vi "Current EXE File Path.vi"(8 "error in (no error)":errorcluster) -> (0 "error out":errorcluster, 3 "Current EXE Path":path)   [LabVIEW 2016, in "SLL Application.lvlib"]
doc: "Provides the current EXE file path. \n\nThis will not work in LabVIEW development environment."
uses:
  SLL Application.lvlib
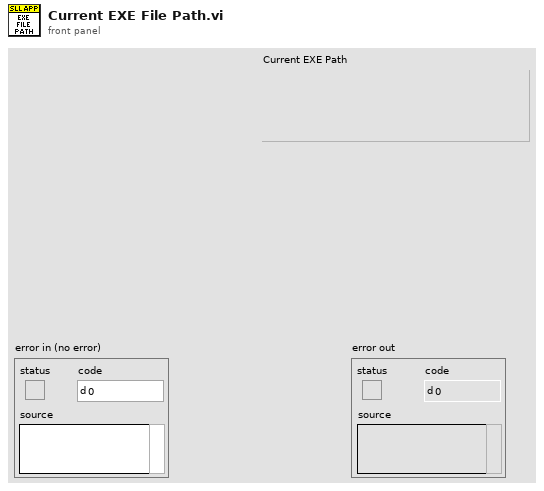
[diagram p1: front panel]
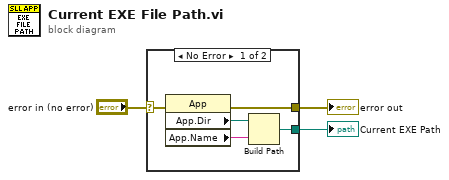
[diagram p0: block diagram]
diagram:
  n1 = case shown="No Error" "error in (no error)" {
    selector: "error in (no error)" -> [w5 w9]
    tunnel: [w6 _] -> w3
    tunnel: [w4 w9] -> w1
    frame No Error {
      n2 = property class="App"(error in=w5) -> (error out=w4:errorcluster, "App.Dir"=w7:path, "App.Name"=w8:string)  [unwired: 1 in, 1 out]
      n3 = Build Path(base path=w7, name or relative path=w8) -> (appended path=w6:path)
    }
    frame Error {
    }
  }
  "error out" <- w1
  "Current EXE Path" <- w3
